vi "MGCC_FntStaMach_Visualization_OpalRT_demo_EvanEdit_v2.vi"() -> ()   [LabVIEW 2016]
panel:
  out "Angle Difference\n0102":dbl format="%#.4f"
  out "Angle Difference\n0405":dbl format="%#.4f"
  out "Angle Difference\n0304":dbl format="%#.4f"
  out "Angle Difference\n0307":dbl format="%#.4f"
  out "Angle Difference\n0709":dbl format="%#.4f"
  out "Angle Difference\n1011":dbl format="%#.4f"
  out "L3":bool
  out "L2":bool
  in  "PV Mode":i32(knob) scale=0.0..2.0
  out "2":cluster{dbl[], dbl[]}(graph)
  out "5":cluster{dbl[], dbl[]}(graph)
  out "4":cluster{dbl[], dbl[]}(graph)
  out "8":cluster{dbl[], dbl[]}(graph)
  out "9":cluster{dbl[], dbl[]}(graph)
  out "11":cluster{dbl[], dbl[]}(graph)
  in  "Stop":bool
  in  "RESET":bool
  out "PV Forecast":dbl[](graph)
  out "3":cluster{dbl[], dbl[]}(graph)
  out "7":cluster{dbl[], dbl[]}(graph)
  out "10":cluster{dbl[], dbl[]}(graph)
  out "13":cluster{dbl[], dbl[]}(graph)
  out "14":cluster{dbl[], dbl[]}(graph)
  out "6":cluster{dbl[], dbl[]}(graph)
  out "1":cluster{dbl[], dbl[]}(graph)
  in  "Tab Control 2":T1(tab)
  out "Loads Power":dbl(graph)
  out "Loads Power":dbl(graph)
  out "Loads Power":dbl(graph)
  out "Loads Power":dbl(graph)
  out "Loads Power":dbl(graph)
  out "Loads Power":dbl(graph)
  out "Loads Power":dbl(graph)
  out "Loads Power":dbl(graph)
  out "Loads Power":dbl(graph)
  in  "Tab Control":T1(tab)
  out "Voltage":dbl(graph)
  out "Voltage":dbl(graph)
  out "Voltage":dbl(graph)
  out "Voltage":dbl(graph)
  out "Voltage":dbl(graph)
  out "Voltage":dbl(graph)
  out "Voltage":dbl(graph)
  out "Voltage":dbl(graph)
  out "Voltage":dbl(graph)
  out "Reactive power control":bool
  out "Active power control":bool
  out "Communication":bool
  out "Reactive power control":bool
  out "Active power control":bool
  out "Resynchronization":bool
  out "Communication":bool
  in  "Island 3":bool
  in  "Island 2":bool
  in  "Island":bool
  in  "Ready for STD":bool
  in  "Recon cmd":bool
  in  "BKS cmd":bool
  in  "island cmd":bool
  out "Angle Difference\n1114":dbl format="%#.4f"
  out "Angle Difference\n0910":dbl format="%#.4f"
  out "Angle Difference\n0406":dbl format="%#.4f"
  out "Angle Difference\n 0203":dbl format="%#.4f"
  out "BESS LC":bool
  out "PV LC":bool
  out "Model Mgmt.":bool
  out "PV Forecasting":bool
  out "Load Forecasting":bool
  out "PQ Balance":bool
  out "Black Start":bool
  out "Data Logging":bool
  out "Communication":bool
  out "State Estimation":bool
  out "Energy Mgmt.":bool
  out "SOC Tank":dbl(slide) scale=0.0..1.0
  out "S1114":bool
  out "S1011":bool
  out "S1012":bool
  out "S1013":bool
  out "S0910":bool
  out "S0708":bool
  out "S0709":bool
  out "S0307":bool
  out "S0304":bool
  out "S0406":bool
  out "S0405":bool
  out "S0203":bool
  out "S0102":bool
  out "W11":bool
  out "W8":bool
  out "L11":bool
  out "W12":bool
  out "L10":bool
  out "L7":bool
  out "L9":bool
  out "W7":bool
  out "L8":bool
  out "L4":bool
  out "L5":bool
  out "W6":bool
  out "W3":bool
  out "W2":bool
  out "Battery Output":dbl format="%#_4f"
  out "Battery SOC":dbl format="%#_4f"
  in  "PV-12":dbl(slide) scale=0.0..2.0
  out "PV Power Output":dbl format="%#_6f"
  out "W4":bool
  out "Current State":string
  out "Sources Power":T2(graph)
  out "Frequency":T3(graph)
  out "W9":bool
  # "Demo: Controller for Flexible Microgrid"
  # "Battery Local Controller"
  # "Microgrid Central\nController"
  # "G-6"
  # "G-14"
  # "G-1"
  # "PV Local Controller"
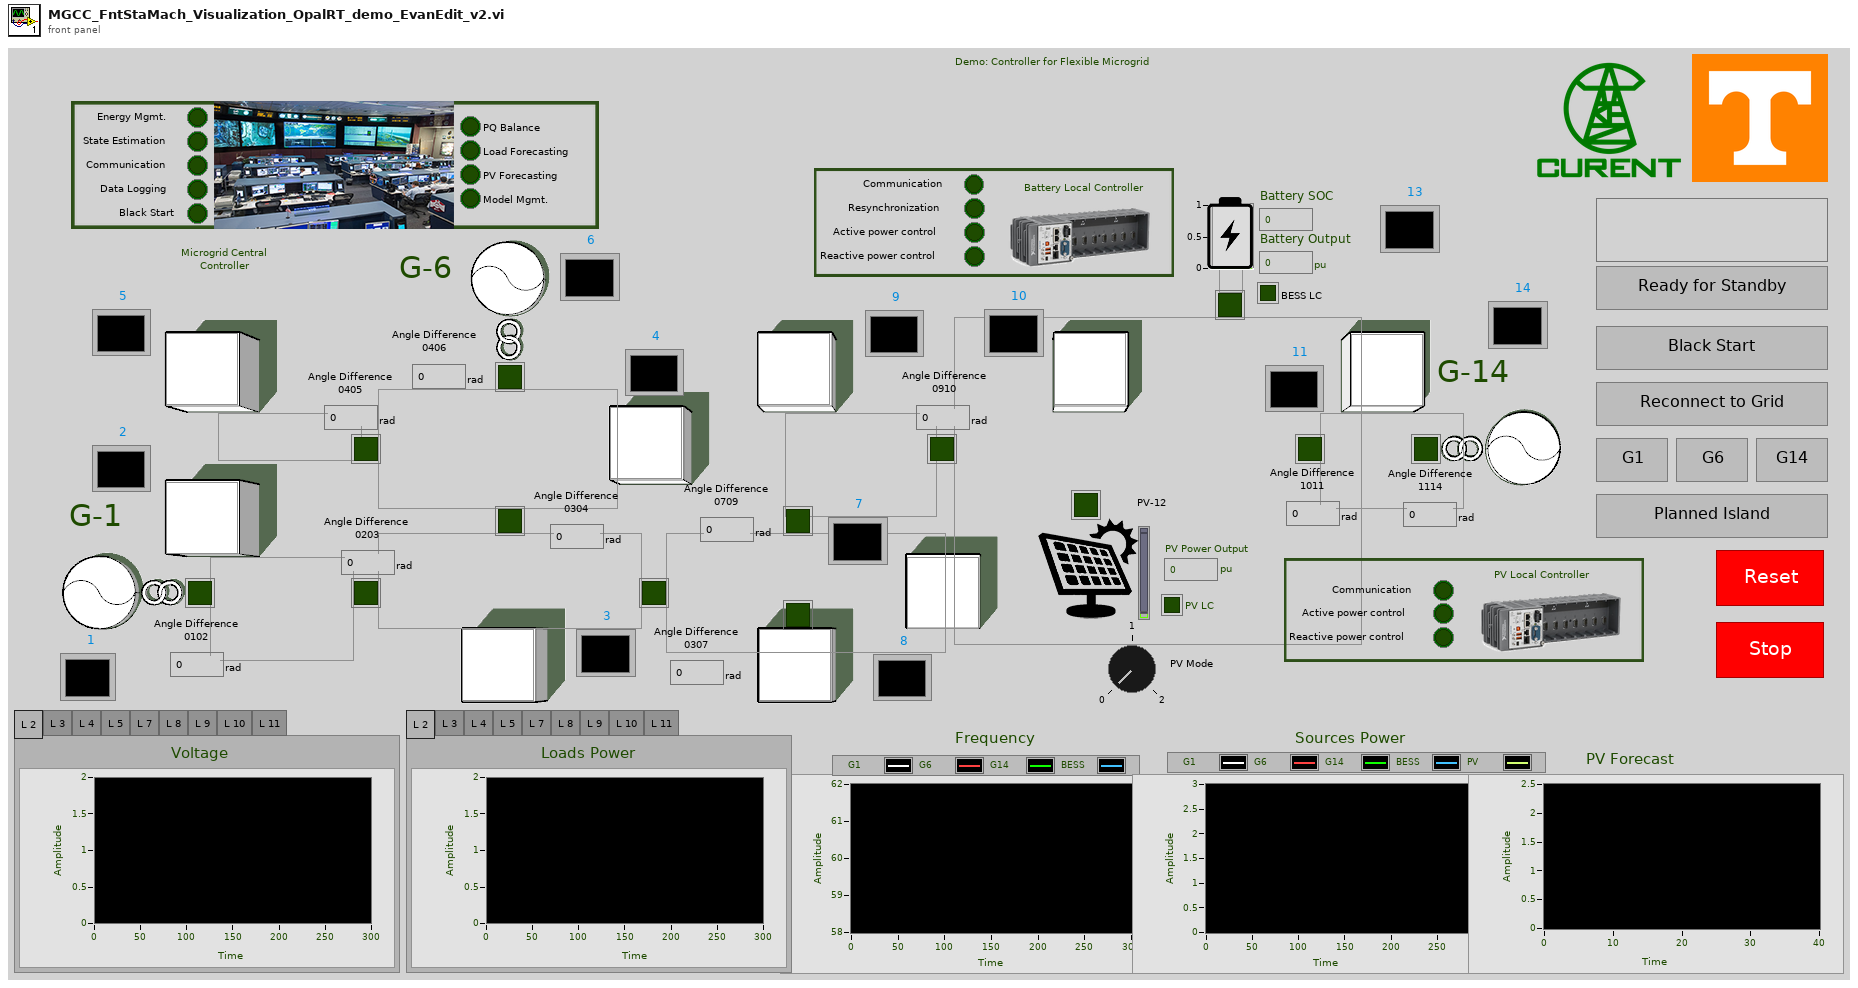
[diagram p1: front panel]
types:
  T1 = enum32{"L 2", "L 3", "L 4", "L 5", "L 7", "L 8", "L 9", "L 10", "L 11"}
  T2 = cluster{"Double":dbl, "Double":dbl, "Double":dbl, "Double":dbl, "Double":dbl}
  T3 = cluster{"Double":dbl, "Double":dbl, "Double":dbl, "Double":dbl}
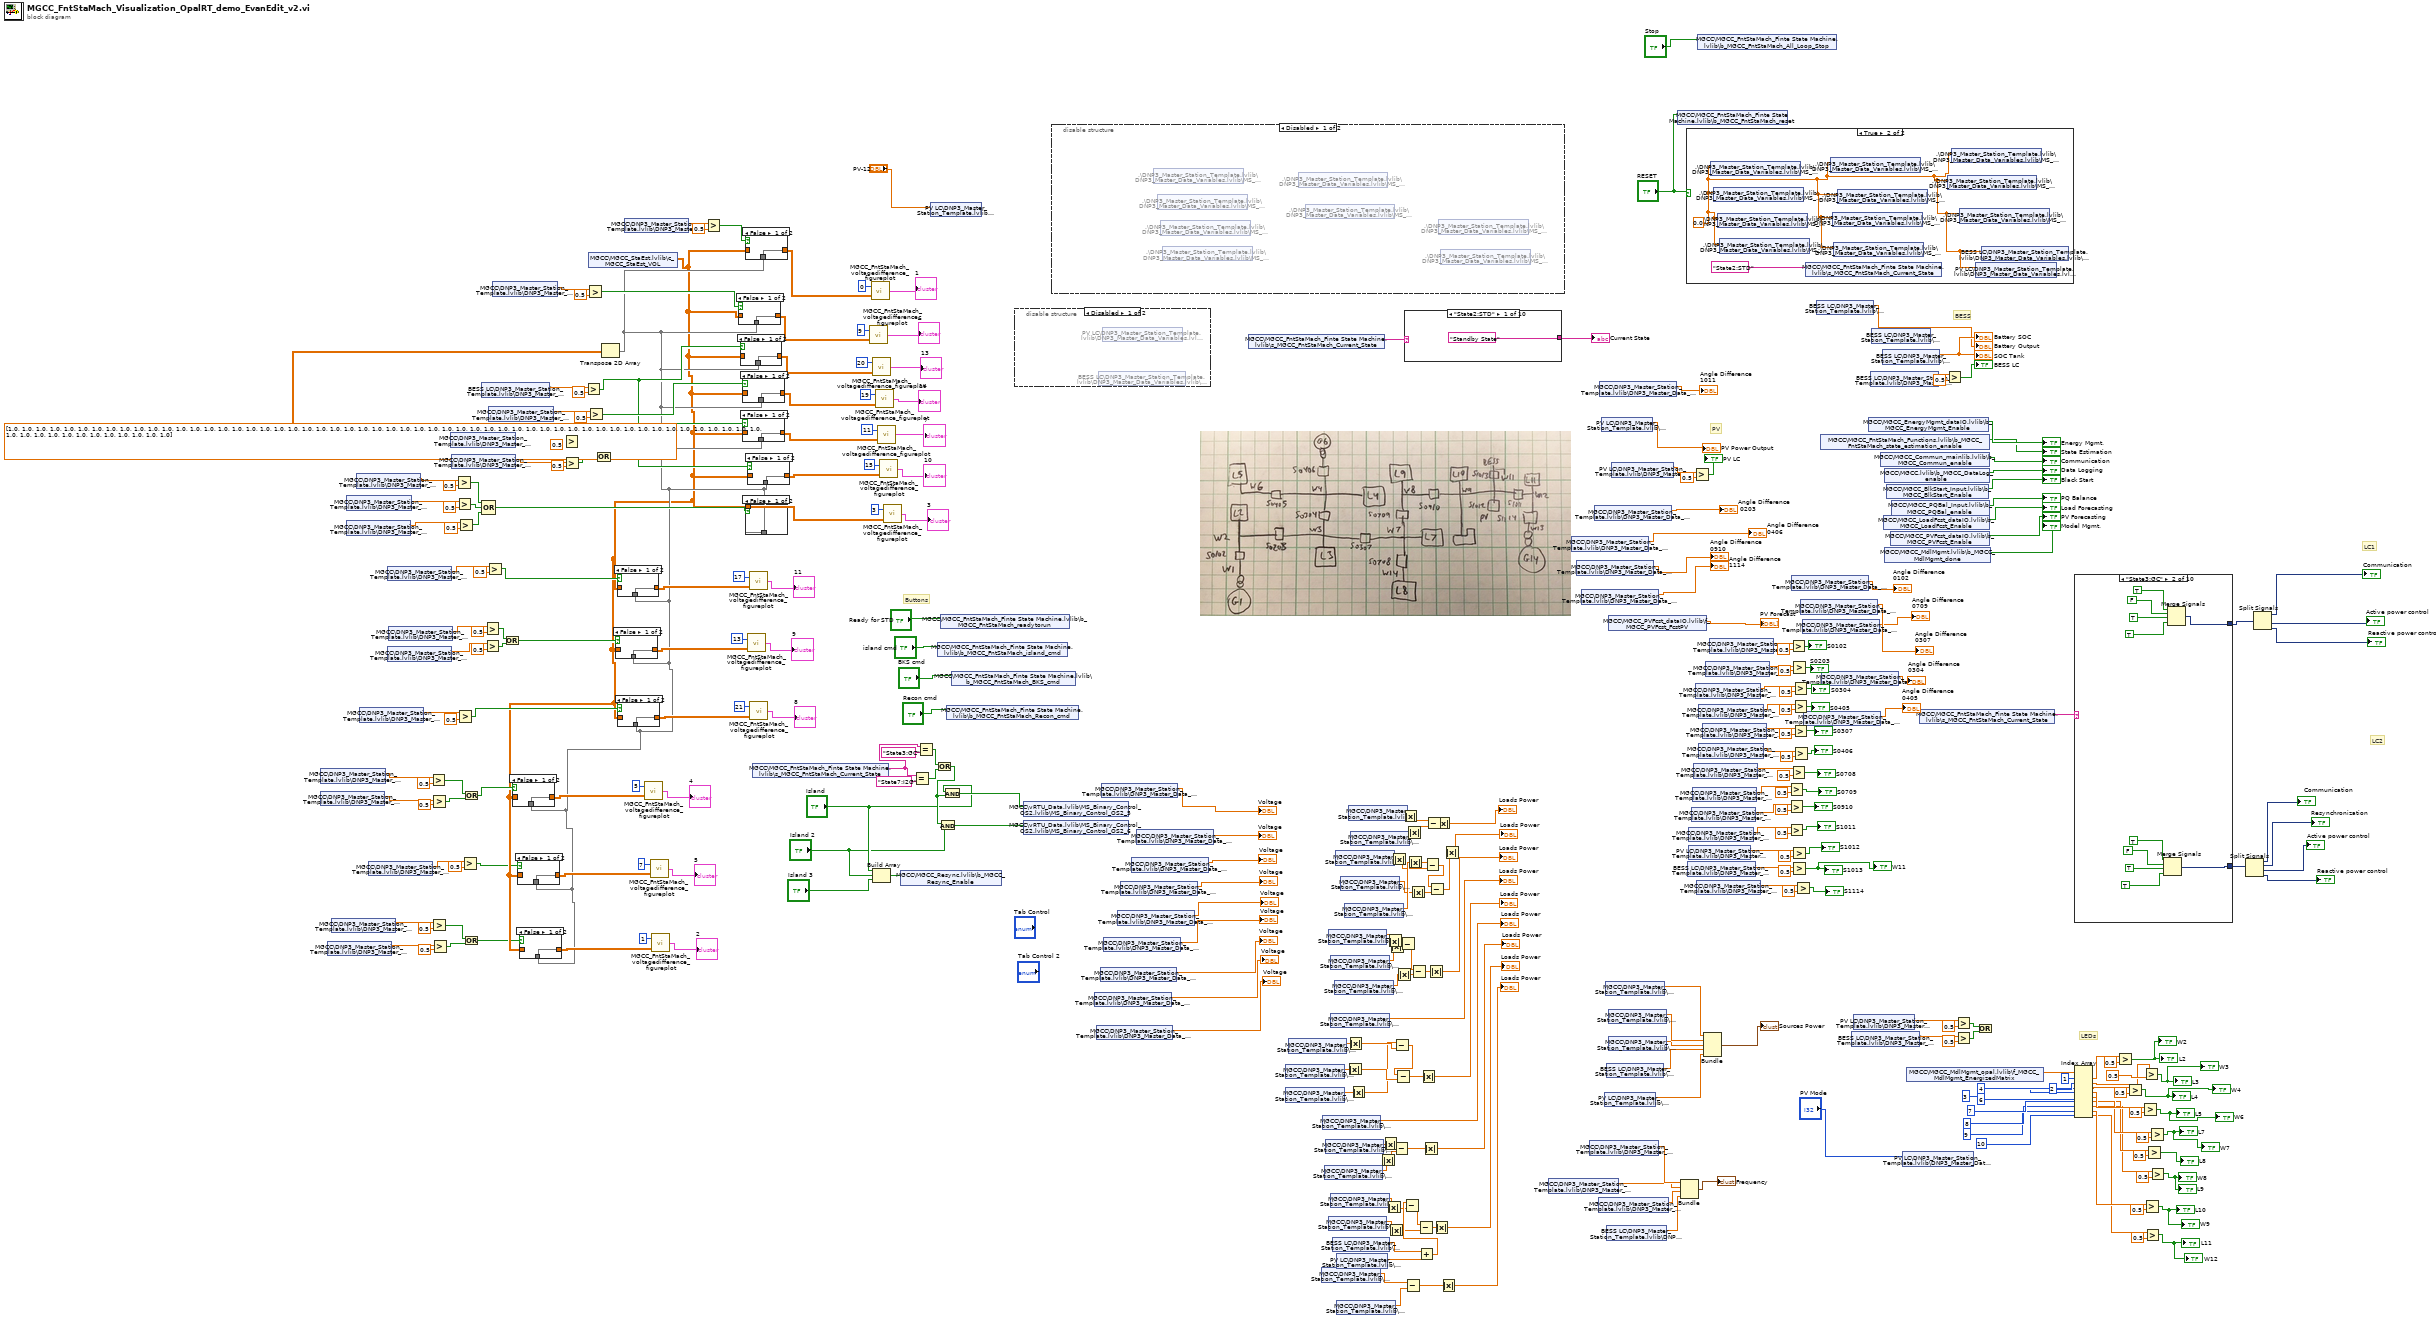
[diagram p0: block diagram]
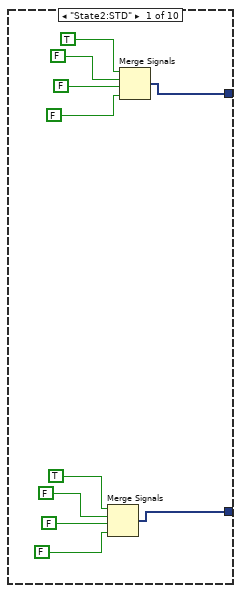
[diagram p2: hidden frame]
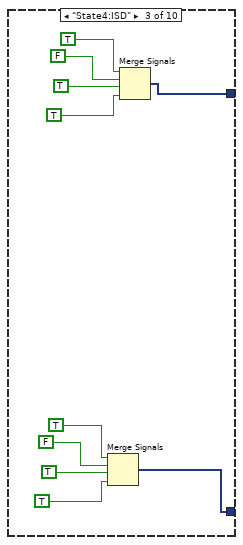
[diagram p3: hidden frame]
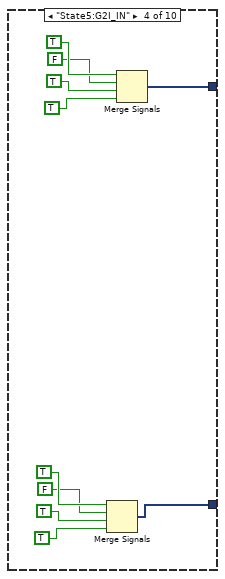
[diagram p4: hidden frame]
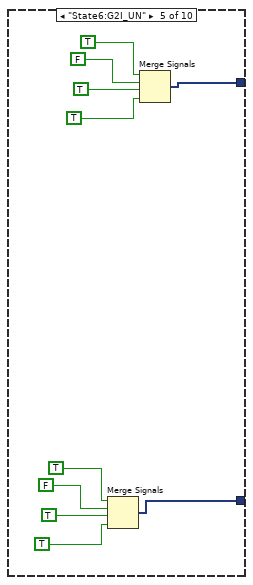
[diagram p5: hidden frame]
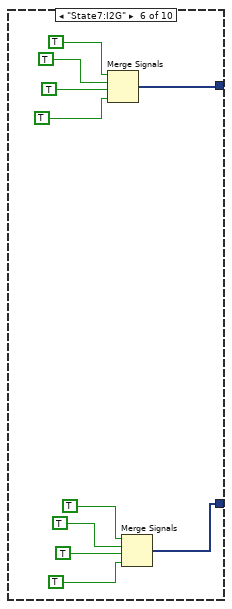
[diagram p6: hidden frame]
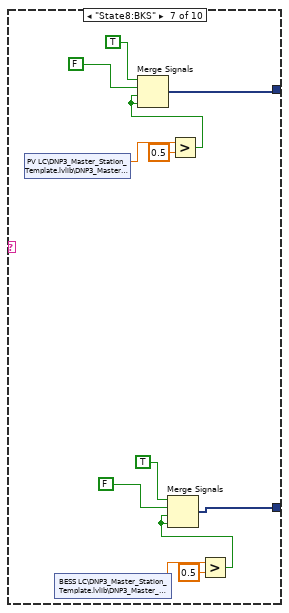
[diagram p7: hidden frame]
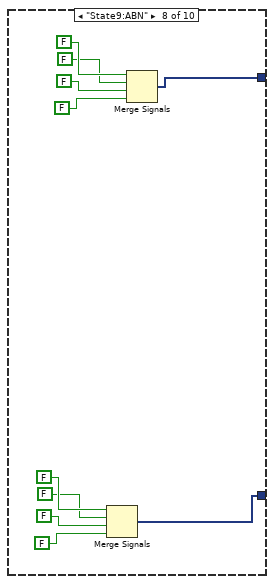
[diagram p8: hidden frame]
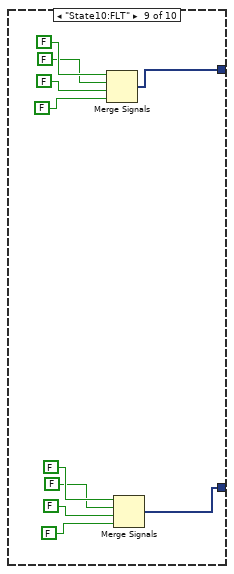
[diagram p9: hidden frame]
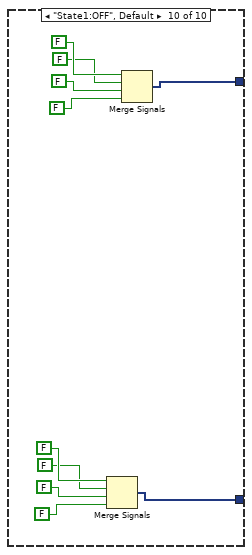
[diagram p10: hidden frame]
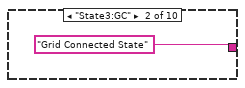
[diagram p18: hidden frame]
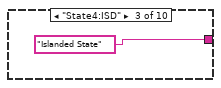
[diagram p19: hidden frame]
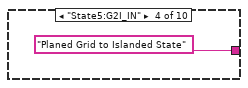
[diagram p20: hidden frame]
diagram:
  # "LC1"
  # "LC2"
  # "PV"
  # "BESS"
  # "Buttons"
  # "LEDs"
  n1 = shared-variable "MGCC\\DNP3_Master_Station_Template.lvlib\\DNP3_Master_Data_Variables.lvlib\\MS_Analog_Status.lvlib\\S0406-status"() -> (w117:dbl)  [unwired: 1 in, 1 out]
  n2 = shared-variable "MGCC\\DNP3_Master_Station_Template.lvlib\\DNP3_Master_Data_Variables.lvlib\\MS_Analog_Status.lvlib\\S0304-status"() -> (w118:dbl)  [unwired: 1 in, 1 out]
  n3 = shared-variable "MGCC\\DNP3_Master_Station_Template.lvlib\\DNP3_Master_Data_Variables.lvlib\\MS_Analog_Status.lvlib\\S0203-status"() -> (w101:dbl)  [unwired: 1 in, 1 out]
  n4 = shared-variable "MGCC\\DNP3_Master_Station_Template.lvlib\\DNP3_Master_Data_Variables.lvlib\\MS_Analog_Status.lvlib\\S0102-status"() -> (w102:dbl)  [unwired: 1 in, 1 out]
  n5 = shared-variable "MGCC\\DNP3_Master_Station_Template.lvlib\\DNP3_Master_Data_Variables.lvlib\\MS_Analog_Status.lvlib\\S0307-status"() -> (w159:dbl)  [unwired: 1 in, 1 out]
  n6 = shared-variable "MGCC\\DNP3_Master_Station_Template.lvlib\\DNP3_Master_Data_Variables.lvlib\\MS_Analog_Status.lvlib\\S0304-status"() -> (w160:dbl)  [unwired: 1 in, 1 out]
  n7 = shared-variable "MGCC\\DNP3_Master_Station_Template.lvlib\\DNP3_Master_Data_Variables.lvlib\\MS_Analog_Status.lvlib\\S0203-status"() -> (w161:dbl)  [unwired: 1 in, 1 out]
  n8 = shared-variable "MGCC\\DNP3_Master_Station_Template.lvlib\\DNP3_Master_Data_Variables.lvlib\\MS_Analog_Status.lvlib\\S0708-status"() -> (w124:dbl)  [unwired: 1 in, 1 out]
  n9 = shared-variable "MGCC\\DNP3_Master_Station_Template.lvlib\\DNP3_Master_Data_Variables.lvlib\\MS_Analog_Status.lvlib\\S0405-status"() -> (w106:dbl)  [unwired: 1 in, 1 out]
  n10 = shared-variable "MGCC\\DNP3_Master_Station_Template.lvlib\\DNP3_Master_Data_Variables.lvlib\\MS_Analog_Status.lvlib\\S1011-status"() -> (w143:dbl)  [unwired: 1 in, 1 out]
  n11 = shared-variable "MGCC\\DNP3_Master_Station_Template.lvlib\\DNP3_Master_Data_Variables.lvlib\\MS_Analog_Status.lvlib\\S0910-status"() -> (w135:dbl)  [unwired: 1 in, 1 out]
  n12 = shared-variable "MGCC\\DNP3_Master_Station_Template.lvlib\\DNP3_Master_Data_Variables.lvlib\\MS_Analog_Status.lvlib\\S0709-status"() -> (w136:dbl)  [unwired: 1 in, 1 out]
  n13 = Greater?(x=w118, y=0.5) -> (0:w120:bool)
  n14 = Greater?(x=w117, y=0.5) -> (0:w119:bool)
  n15 = Greater?(x=w102, y=0.5) -> (0:w100:bool)
  n16 = Greater?(x=w101, y=0.5) -> (0:w99:bool)
  n17 = shared-variable "MGCC\\DNP3_Master_Station_Template.lvlib\\DNP3_Master_Data_Variables.lvlib\\MS_Analog_Status.lvlib\\S0307-status"() -> (w171:dbl)  [unwired: 1 in, 1 out]
  n18 = shared-variable "MGCC\\DNP3_Master_Station_Template.lvlib\\DNP3_Master_Data_Variables.lvlib\\MS_Analog_Status.lvlib\\S0709-status"() -> (w170:dbl)  [unwired: 1 in, 1 out]
  n19 = Greater?(x=w161, y=0.5) -> (0:w158:bool)
  n20 = Greater?(x=w160, y=0.5) -> (0:w157:bool)
  n21 = Greater?(x=w124, y=0.5) -> (0:w123:bool)
  n22 = Greater?(x=w159, y=0.5) -> (0:w156:bool)
  n23 = Greater?(x=w106, y=0.5) -> (0:w105:bool)
  n24 = Or(x=w120, y=w119) -> (x .or. y?=w116:bool)
  n25 = Or(x=w100, y=w99) -> (x .or. y?=w98:bool)
  n26 = shared-variable "BESS LC\\DNP3_Master_Station_Template.lvlib\\DNP3_Master_Data_Variables.lvlib\\MS_Analog_Status.lvlib\\BESS-STATUS"() -> (w183:dbl)  [unwired: 1 in, 1 out]
  n27 = Compound Arithmetic op=OR(w158, w157, w156) -> (w155:bool)
  n28 = Greater?(x=w136, y=0.5) -> (0:w134:bool)
  n29 = Greater?(x=w135, y=0.5) -> (0:w133:bool)
  n30 = Greater?(x=w143, y=0.5) -> (0:w142:bool)
  n31 = shared-variable "MGCC\\DNP3_Master_Station_Template.lvlib\\DNP3_Master_Data_Variables.lvlib\\MS_Analog_Status.lvlib\\S1114-status"() -> (w177:dbl)  [unwired: 1 in, 1 out]
  n32 = shared-variable "MGCC\\DNP3_Master_Station_Template.lvlib\\DNP3_Master_Data_Variables.lvlib\\MS_Analog_Status.lvlib\\S0406-status"() -> (w186:dbl)  [unwired: 1 in, 1 out]
  n33 = Or(x=w134, y=w133) -> (x .or. y?=w132:bool)
  n34 = Greater?(x=w171, y=0.5) -> (0:w173:bool)
  n35 = Greater?(x=w170, y=0.5) -> (0:w172:bool)
  n36 = Greater?(x=w183, y=0.5) -> (0:w168:bool)
  n37 = Greater?(x=w186, y=0.5) -> (0:w185:bool)
  n38 = Greater?(x=w177, y=0.5) -> (0:w176:bool)
  n39 = shared-variable "MGCC\\MGCC_StaEst.lvlib\\c_MGCC_StaEst_VOL"() -> (w108:cdb[][])  [unwired: 1 in, 1 out]
  n40 = Or(x=w173, y=w172) -> (x .or. y?=w169:bool)
  n41 = Transpose 2D Array(2D array=dbl[][] [[1.0, 1.0, 1.0, 1.0, 1.0, 1.0, 1.0, 1.0, 1.0, 1.0, 1.0, 1.0, 1.0, 1.0, 1.0, 1.0, 1.0, 1.0, 1.0, 1.0, 1.0, 1.0], [1.0, 1.0, 1.0, 1.0, 1.0, 1.0, 1.0, 1.0, 1.0, 1.0, 1.0, 1.0, 1.0, 1.0, 1.0, 1.0, 1.0, 1.0, 1.0, 1.0, 1.0, 1.0], [1.0, 1.0, 1.0, 1.0, 1.0, 1.0, 1.0, 1.0, 1.0, 1.0, 1.0, 1.0, 1.0, 1.0, 1.0, 1.0, 1.0, 1.0, 1.0, 1.0, 1.0, 1.0]] ("lower limit")) -> (transposed array=w109:dbl[][])
  n42 = case shown="False" w116 {
    tunnel: w108 -> [_ w321]
    tunnel: [w320 w321] -> w126
    tunnel: w109 -> [w320 _]
    frame False {
    }
    frame True {
    }
  }
  n43 = case shown="False" w105 {
    tunnel: w108 -> [_ w323]
    tunnel: [w322 w323] -> w113
    tunnel: w109 -> [w322 _]
    frame False {
    }
    frame True {
    }
  }
  n44 = case shown="False" w98 {
    tunnel: w108 -> [_ w325]
    tunnel: [w324 w325] -> w110
    tunnel: w109 -> [w324 _]
    frame False {
    }
    frame True {
    }
  }
  n45 = case shown="False" w132 {
    tunnel: w108 -> [_ w327]
    tunnel: [w326 w327] -> w139
    tunnel: w109 -> [w326 _]
    frame False {
    }
    frame True {
    }
  }
  n46 = case shown="False" w142 {
    tunnel: w108 -> [_ w329]
    tunnel: [w328 w329] -> w145
    tunnel: w109 -> [w328 _]
    frame False {
    }
    frame True {
    }
  }
  n47 = case shown="False" w123 {
    tunnel: w108 -> [_ w331]
    tunnel: [w330 w331] -> w129
    tunnel: w109 -> [w330 _]
    frame False {
    }
    frame True {
    }
  }
  n48 = shared-variable "MGCC\\DNP3_Master_Station_Template.lvlib\\DNP3_Master_Data_Variables.lvlib\\MS_Analog_Status.lvlib\\S0102-status"() -> (w190:dbl)  [unwired: 1 in, 1 out]
  n49 = call "MGCC_FntStaMach_voltagedifference_figureplot.vi"("array"=w126, "index (row)"=5) -> ("output cluster"=→"4":cluster{dbl[], dbl[]})
  n50 = call "MGCC_FntStaMach_voltagedifference_figureplot.vi"("array"=w113, "index (row)"=7) -> ("output cluster"=→"5":cluster{dbl[], dbl[]})
  n51 = call "MGCC_FntStaMach_voltagedifference_figureplot.vi"("array"=w110, "index (row)"=1) -> ("output cluster"=→"2":cluster{dbl[], dbl[]})
  n52 = Greater?(x=w190, y=0.5) -> (0:w189:bool)
  n53 = case shown="False" w185 {
    tunnel: w108 -> [_ w333]
    tunnel: [w332 w333] -> w188
    tunnel: w109 -> [w332 _]
    frame False {
    }
    frame True {
    }
  }
  n54 = case shown="False" w168 {
    tunnel: w108 -> [_ w335]
    tunnel: [w334 w335] -> w182
    tunnel: w109 -> [w334 _]
    frame False {
    }
    frame True {
    }
  }
  n55 = case shown="False" w176 {
    tunnel: w108 -> [_ w337]
    tunnel: [w336 w337] -> w181
    tunnel: w109 -> [w336 _]
    frame False {
    }
    frame True {
    }
  }
  n56 = case shown="False" w169 {
    tunnel: w108 -> [_ w339]
    tunnel: [w338 w339] -> w180
    tunnel: w109 -> [w338 _]
    frame False {
    }
    frame True {
    }
  }
  n57 = case shown="False" w189 {
    tunnel: w108 -> [_ w341]
    tunnel: [w340 w341] -> w192
    tunnel: w109 -> [w340 _]
    frame False {
    }
    frame True {
    }
  }
  n58 = case shown="False" w155 {
    tunnel: w108 -> [_ w343]
    tunnel: [w342 w343] -> w165
    tunnel: w109 -> [w342 _]
    frame False {
    }
    frame True {
    }
  }
  n59 = case shown="False" w168 {
    tunnel: w108 -> [_ w345]
    tunnel: [w344 w345] -> w179
    tunnel: w109 -> [w344 _]
    frame False {
    }
    frame True {
    }
  }
  n60 = call "MGCC_FntStaMach_voltagedifference_figureplot.vi"("array"=w139, "index (row)"=13) -> ("output cluster"=→"9":cluster{dbl[], dbl[]})
  n61 = call "MGCC_FntStaMach_voltagedifference_figureplot.vi"("array"=w145, "index (row)"=17) -> ("output cluster"=→"11":cluster{dbl[], dbl[]})
  n62 = call "MGCC_FntStaMach_voltagedifference_figureplot.vi"("array"=w129, "index (row)"=21) -> ("output cluster"=→"8":cluster{dbl[], dbl[]})
  n63 = shared-variable "MGCC\\MGCC_FntStaMach_Finte State Machine.lvlib\\s_MGCC_FntStaMach_Current_State"() -> (w206:string)  [unwired: 1 in, 1 out]
  n64 = call "MGCC_FntStaMach_voltagedifference_figureplot.vi"("array"=w188, "index (row)"=9) -> ("output cluster"=→"6":cluster{dbl[], dbl[]})
  n65 = call "MGCC_FntStaMach_voltagedifference_figureplot.vi"("array"=w192, "index (row)"=0) -> ("output cluster"=→"1":cluster{dbl[], dbl[]})
  n66 = call "MGCC_FntStaMach_voltagedifference_figureplot.vi"("array"=w182, "index (row)"=20) -> ("output cluster"=→"13":cluster{dbl[], dbl[]})
  n67 = Build Array("Island", "Island 2", "Island 3") -> (w79:bool[])
  n68 = call "MGCC_FntStaMach_voltagedifference_figureplot.vi"("array"=w181, "index (row)"=19) -> ("output cluster"=→"14":cluster{dbl[], dbl[]})
  n69 = call "MGCC_FntStaMach_voltagedifference_figureplot.vi"("array"=w180, "index (row)"=11) -> ("output cluster"=→"7":cluster{dbl[], dbl[]})
  n70 = call "MGCC_FntStaMach_voltagedifference_figureplot.vi"("array"=w179, "index (row)"=15) -> ("output cluster"=→"10":cluster{dbl[], dbl[]})
  n71 = call "MGCC_FntStaMach_voltagedifference_figureplot.vi"("array"=w165, "index (row)"=3) -> ("output cluster"=→"3":cluster{dbl[], dbl[]})
  n72 = shared-variable "MGCC\\MGCC_Resync.lvlib\\b_MGCC_Resync_Enable"(w79) -> ()  [unwired: 1 in, 1 out]
  n73 = Equal?(x=w206, y="State7:I2G") -> (x = y?=w297:bool)
  n74 = Equal?(x=w206, y="State3:GC") -> (x = y?=w296:bool)
  n75 = shared-variable "PV LC\\DNP3_Master_Station_Template.lvlib\\DNP3_Master_Data_Variables.lvlib\\MS_Analog_Control.lvlib\\PV-APC"("PV-12") -> ()  [unwired: 1 in, 1 out]
  n76 = Or(x=w296, y=w297) -> (x .or. y?=w295:bool)
  n77 = shared-variable "MGCC\\MGCC_FntStaMach_Finte State Machine.lvlib\\b_MGCC_FntStaMach_island_cmd"("island cmd") -> ()  [unwired: 1 in, 1 out]
  n78 = And(x=w295, y="Island 2") -> (x .and. y?=w293:bool)
  n79 = shared-variable "MGCC\\MGCC_FntStaMach_Finte State Machine.lvlib\\b_MGCC_FntStaMach_readytorun"("Ready for STD") -> ()  [unwired: 1 in, 1 out]
  n80 = And(x="Island", y=w295) -> (x .and. y?=w294:bool)
  n81 = shared-variable "MGCC\\MGCC_FntStaMach_Finte State Machine.lvlib\\b_MGCC_FntStaMach_Recon_cmd"("Recon cmd") -> ()  [unwired: 1 in, 1 out]
  n82 = shared-variable "MGCC\\MGCC_FntStaMach_Finte State Machine.lvlib\\b_MGCC_FntStaMach_BKS_cmd"("BKS cmd") -> ()  [unwired: 1 in, 1 out]
  n83 = disable-structure shown="Disabled" {
    frame Disabled {
      n84 = shared-variable "BESS LC\\DNP3_Master_Station_Template.lvlib\\DNP3_Master_Data_Variables.lvlib\\MS_Analog_Control.lvlib\\BESS-STATUS-CTRL"() -> (w347:dbl)  [unwired: 1 in, 1 out]
      n85 = shared-variable "PV LC\\DNP3_Master_Station_Template.lvlib\\DNP3_Master_Data_Variables.lvlib\\MS_Analog_Control.lvlib\\PV-STATUS-CTRL"() -> (w346:dbl)  [unwired: 1 in, 1 out]
    }
    frame Enabled {
    }
  }
  n86 = shared-variable "MGCC\\vRTU_Data.lvlib\\MS_Binary_Control_OS2.lvlib\\MS_Binary_Control_OS2_5"(w294) -> ()  [unwired: 1 in, 1 out]
  n87 = shared-variable "MGCC\\vRTU_Data.lvlib\\MS_Binary_Control_OS2.lvlib\\MS_Binary_Control_OS2_6"(w293) -> ()  [unwired: 1 in, 1 out]
  n88 = disable-structure shown="Disabled" {
    frame Disabled {
      n89 = shared-variable ".\\DNP3_Master_Station_Template.lvlib\\DNP3_Master_Data_Variables.lvlib\\MS_Analog_Control.lvlib\\S0203-STATUS-CTRL"() -> (w355:dbl)  [unwired: 1 in, 1 out]
      n90 = shared-variable ".\\DNP3_Master_Station_Template.lvlib\\DNP3_Master_Data_Variables.lvlib\\MS_Analog_Control.lvlib\\S0304-STATUS-CTRL"() -> (w354:dbl)  [unwired: 1 in, 1 out]
      n91 = shared-variable ".\\DNP3_Master_Station_Template.lvlib\\DNP3_Master_Data_Variables.lvlib\\MS_Analog_Control.lvlib\\S0307-STATUS-CTRL"() -> (w353:dbl)  [unwired: 1 in, 1 out]
      n92 = shared-variable ".\\DNP3_Master_Station_Template.lvlib\\DNP3_Master_Data_Variables.lvlib\\MS_Analog_Control.lvlib\\S0405-STATUS-CTRL"() -> (w352:dbl)  [unwired: 1 in, 1 out]
      n93 = shared-variable ".\\DNP3_Master_Station_Template.lvlib\\DNP3_Master_Data_Variables.lvlib\\MS_Analog_Control.lvlib\\S0708-STATUS-CTRL"() -> (w351:dbl)  [unwired: 1 in, 1 out]
      n94 = shared-variable ".\\DNP3_Master_Station_Template.lvlib\\DNP3_Master_Data_Variables.lvlib\\MS_Analog_Control.lvlib\\S0709-STATUS-CTRL"() -> (w350:dbl)  [unwired: 1 in, 1 out]
      n95 = shared-variable ".\\DNP3_Master_Station_Template.lvlib\\DNP3_Master_Data_Variables.lvlib\\MS_Analog_Control.lvlib\\S0910-STATUS-CTRL"() -> (w349:dbl)  [unwired: 1 in, 1 out]
      n96 = shared-variable ".\\DNP3_Master_Station_Template.lvlib\\DNP3_Master_Data_Variables.lvlib\\MS_Analog_Control.lvlib\\S1011-STATUS-CTRL"() -> (w348:dbl)  [unwired: 1 in, 1 out]
    }
    frame Enabled {
    }
  }
  n97 = shared-variable "MGCC\\DNP3_Master_Station_Template.lvlib\\DNP3_Master_Data_Variables.lvlib\\MS_Analog_Status.lvlib\\S0910-MAG-A-R"() -> (→"Voltage":dbl)  [unwired: 1 in, 1 out]
  n98 = shared-variable "MGCC\\DNP3_Master_Station_Template.lvlib\\DNP3_Master_Data_Variables.lvlib\\MS_Analog_Status.lvlib\\S1011-MAG-A-R"() -> (→"Voltage":dbl)  [unwired: 1 in, 1 out]
  n99 = shared-variable "MGCC\\DNP3_Master_Station_Template.lvlib\\DNP3_Master_Data_Variables.lvlib\\MS_Analog_Status.lvlib\\S0709-MAG-A-R"() -> (→"Voltage":dbl)  [unwired: 1 in, 1 out]
  n100 = shared-variable "MGCC\\DNP3_Master_Station_Template.lvlib\\DNP3_Master_Data_Variables.lvlib\\MS_Analog_Status.lvlib\\S0102-MAG-A-R"() -> (→"Voltage":dbl)  [unwired: 1 in, 1 out]
  n101 = shared-variable "MGCC\\DNP3_Master_Station_Template.lvlib\\DNP3_Master_Data_Variables.lvlib\\MS_Analog_Status.lvlib\\S0708-MAG-A-R"() -> (→"Voltage":dbl)  [unwired: 1 in, 1 out]
  n102 = shared-variable "MGCC\\DNP3_Master_Station_Template.lvlib\\DNP3_Master_Data_Variables.lvlib\\MS_Analog_Status.lvlib\\S0307-MAG-A-R"() -> (→"Voltage":dbl)  [unwired: 1 in, 1 out]
  n103 = shared-variable "MGCC\\DNP3_Master_Station_Template.lvlib\\DNP3_Master_Data_Variables.lvlib\\MS_Analog_Status.lvlib\\S0405-MAG-A-R"() -> (→"Voltage":dbl)  [unwired: 1 in, 1 out]
  n104 = shared-variable "MGCC\\DNP3_Master_Station_Template.lvlib\\DNP3_Master_Data_Variables.lvlib\\MS_Analog_Status.lvlib\\S0304-MAG-A-R"() -> (→"Voltage":dbl)  [unwired: 1 in, 1 out]
  n105 = shared-variable "MGCC\\DNP3_Master_Station_Template.lvlib\\DNP3_Master_Data_Variables.lvlib\\MS_Analog_Status.lvlib\\S0203-MAG-A-R"() -> (→"Voltage":dbl)  [unwired: 1 in, 1 out]
  n106 = shared-variable "MGCC\\MGCC_FntStaMach_Finte State Machine.lvlib\\s_MGCC_FntStaMach_Current_State"() -> (w152:string)  [unwired: 1 in, 1 out]
  n107 = shared-variable "MGCC\\DNP3_Master_Station_Template.lvlib\\DNP3_Master_Data_Variables.lvlib\\MS_Analog_Status.lvlib\\S0708-APF"() -> (w26:dbl)  [unwired: 1 in, 1 out]
  n108 = shared-variable "MGCC\\DNP3_Master_Station_Template.lvlib\\DNP3_Master_Data_Variables.lvlib\\MS_Analog_Status.lvlib\\S0709-APF"() -> (w28:dbl)  [unwired: 1 in, 1 out]
  n109 = shared-variable "MGCC\\DNP3_Master_Station_Template.lvlib\\DNP3_Master_Data_Variables.lvlib\\MS_Analog_Status.lvlib\\S0307-APF"() -> (w27:dbl)  [unwired: 1 in, 1 out]
  n110 = shared-variable "MGCC\\DNP3_Master_Station_Template.lvlib\\DNP3_Master_Data_Variables.lvlib\\MS_Analog_Status.lvlib\\S1011-APF"() -> (w265:dbl)  [unwired: 1 in, 1 out]
  n111 = shared-variable "MGCC\\DNP3_Master_Station_Template.lvlib\\DNP3_Master_Data_Variables.lvlib\\MS_Analog_Status.lvlib\\S0708-APF"() -> (→"Loads Power":dbl)  [unwired: 1 in, 1 out]
  n112 = shared-variable "MGCC\\DNP3_Master_Station_Template.lvlib\\DNP3_Master_Data_Variables.lvlib\\MS_Analog_Status.lvlib\\S0910-APF"() -> (w268:dbl)  [unwired: 1 in, 1 out]
  n113 = shared-variable "MGCC\\DNP3_Master_Station_Template.lvlib\\DNP3_Master_Data_Variables.lvlib\\MS_Analog_Status.lvlib\\S0709-APF"() -> (w269:dbl)  [unwired: 1 in, 1 out]
  n114 = shared-variable "MGCC\\DNP3_Master_Station_Template.lvlib\\DNP3_Master_Data_Variables.lvlib\\MS_Analog_Status.lvlib\\S0304-APF"() -> (w278:dbl)  [unwired: 1 in, 1 out]
  n115 = shared-variable "MGCC\\DNP3_Master_Station_Template.lvlib\\DNP3_Master_Data_Variables.lvlib\\MS_Analog_Status.lvlib\\S1011-APF"() -> (w11:dbl)  [unwired: 1 in, 1 out]
  n116 = shared-variable "MGCC\\DNP3_Master_Station_Template.lvlib\\DNP3_Master_Data_Variables.lvlib\\MS_Analog_Status.lvlib\\S0405-APF"() -> (w277:dbl)  [unwired: 1 in, 1 out]
  n117 = shared-variable "MGCC\\DNP3_Master_Station_Template.lvlib\\DNP3_Master_Data_Variables.lvlib\\MS_Analog_Status.lvlib\\S0405-APF"() -> (→"Loads Power":dbl)  [unwired: 1 in, 1 out]
  n118 = shared-variable "MGCC\\DNP3_Master_Station_Template.lvlib\\DNP3_Master_Data_Variables.lvlib\\MS_Analog_Status.lvlib\\S0910-APF"() -> (w12:dbl)  [unwired: 1 in, 1 out]
  n119 = shared-variable "BESS LC\\DNP3_Master_Station_Template.lvlib\\DNP3_Master_Data_Variables.lvlib\\MS_Analog_Status.lvlib\\BESS-APO"() -> (w15:dbl)  [unwired: 1 in, 1 out]
  n120 = shared-variable "MGCC\\DNP3_Master_Station_Template.lvlib\\DNP3_Master_Data_Variables.lvlib\\MS_Analog_Status.lvlib\\S0406-APF"() -> (w275:dbl)  [unwired: 1 in, 1 out]
  n121 = shared-variable "MGCC\\DNP3_Master_Station_Template.lvlib\\DNP3_Master_Data_Variables.lvlib\\MS_Analog_Status.lvlib\\S0203-APF"() -> (w36:dbl)  [unwired: 1 in, 1 out]
  n122 = shared-variable "PV LC\\DNP3_Master_Station_Template.lvlib\\DNP3_Master_Data_Variables.lvlib\\MS_Analog_Status.lvlib\\PV-APO"() -> (w14:dbl)  [unwired: 1 in, 1 out]
  n123 = shared-variable "MGCC\\DNP3_Master_Station_Template.lvlib\\DNP3_Master_Data_Variables.lvlib\\MS_Analog_Status.lvlib\\S1114-APF"() -> (w264:dbl)  [unwired: 1 in, 1 out]
  n124 = shared-variable "MGCC\\DNP3_Master_Station_Template.lvlib\\DNP3_Master_Data_Variables.lvlib\\MS_Analog_Status.lvlib\\S0304-APF"() -> (w35:dbl)  [unwired: 1 in, 1 out]
  n125 = shared-variable "MGCC\\DNP3_Master_Station_Template.lvlib\\DNP3_Master_Data_Variables.lvlib\\MS_Analog_Status.lvlib\\S0307-APF"() -> (w37:dbl)  [unwired: 1 in, 1 out]
  n126 = Absolute Value(x=w26) -> (abs(x)=w24:dbl)
  n127 = Absolute Value(x=w27) -> (abs(x)=w25:dbl)
  n128 = shared-variable "MGCC\\DNP3_Master_Station_Template.lvlib\\DNP3_Master_Data_Variables.lvlib\\MS_Analog_Status.lvlib\\S0102-APF"() -> (w283:dbl)  [unwired: 1 in, 1 out]
  n129 = Absolute Value(x=w28) -> (abs(x)=w23:dbl)
  n130 = shared-variable "MGCC\\DNP3_Master_Station_Template.lvlib\\DNP3_Master_Data_Variables.lvlib\\MS_Analog_Status.lvlib\\S0203-APF"() -> (w282:dbl)  [unwired: 1 in, 1 out]
  n131 = Absolute Value(x=w268) -> (abs(x)=w21:dbl)
  n132 = Absolute Value(x=w269) -> (abs(x)=w22:dbl)
  n133 = Absolute Value(x=w12) -> (abs(x)=w10:dbl)
  n134 = Absolute Value(x=w278) -> (abs(x)=w31:dbl)
  n135 = Absolute Value(x=w11) -> (abs(x)=w9:dbl)
  n136 = Absolute Value(x=w277) -> (abs(x)=w30:dbl)
  n137 = Absolute Value(x=w36) -> (abs(x)=w34:dbl)
  n138 = Subtract(x=w22, y=w21) -> (x-y=w267:dbl)
  n139 = Subtract(x=w23, y=w25) -> (x-y=w272:dbl)
  n140 = Subtract(x=w272, y=w24) -> (x-y=w271:dbl)
  n141 = Absolute Value(x=w275) -> (abs(x)=w29:dbl)
  n142 = Subtract(x=w31, y=w30) -> (x-y=w276:dbl)
  n143 = Absolute Value(x=w283) -> (abs(x)=w40:dbl)
  n144 = case shown="\"State2:STD\"" w152 {
    tunnel: ["Standby State" "Grid Connected State" "Islanded State" "Planed Grid to Islanded State" "Unplaned Grid to Islaned State" "Islanded to Grid State" "Black Start State" "Abnormal State" "Fault State" "Off State"] -> w151
    frame "State2:STD" {
    }
    frame "State3:GC" {
    }
    frame "State4:ISD" {
    }
    frame "State5:G2I_IN" {
    }
    frame "State6:G2I_UN" {
    }
    frame "State7:I2G" {
    }
    frame "State8:BKS" {
    }
    frame "State9:ABN" {
    }
    frame "State10:FLT" {
    }
    frame "State1:OFF", Default {
    }
  }
  "Current State" <- w151
  n145 = Subtract(x=w265, y=w264) -> (x-y=w263:dbl)
  n146 = Absolute Value(x=w282) -> (abs(x)=w39:dbl)
  n147 = Absolute Value(x=w37) -> (abs(x)=w33:dbl)
  n148 = Absolute Value(x=w35) -> (abs(x)=w32:dbl)
  n149 = Subtract(x=w276, y=w29) -> (x-y=w274:dbl)
  n150 = Add(x=w15, y=w14) -> (x+y=w13:dbl)
  n151 = Subtract(x=w13, y=w10) -> (x-y=w266:dbl)
  n152 = Subtract(x=w266, y=w9) -> (x-y=w16:dbl)
  n153 = Absolute Value(x=w271) -> (abs(x)=→"Loads Power":dbl)
  n154 = Absolute Value(x=w267) -> (abs(x)=→"Loads Power":dbl)
  n155 = Subtract(x=w33, y=w34) -> (x-y=w280:dbl)
  n156 = Subtract(x=w40, y=w39) -> (x-y=w281:dbl)
  n157 = Absolute Value(x=w274) -> (abs(x)=→"Loads Power":dbl)
  n158 = Subtract(x=w280, y=w32) -> (x-y=w279:dbl)
  n159 = Absolute Value(x=w16) -> (abs(x)=→"Loads Power":dbl)
  n160 = Absolute Value(x=w281) -> (abs(x)=→"Loads Power":dbl)
  n161 = Absolute Value(x=w263) -> (abs(x)=→"Loads Power":dbl)
  n162 = Absolute Value(x=w279) -> (abs(x)=→"Loads Power":dbl)
  n163 = shared-variable "MGCC\\DNP3_Master_Station_Template.lvlib\\DNP3_Master_Data_Variables.lvlib\\MS_Analog_Status.lvlib\\S0406-FREQ-R"() -> (w261:dbl)  [unwired: 1 in, 1 out]
  n164 = shared-variable "MGCC\\DNP3_Master_Station_Template.lvlib\\DNP3_Master_Data_Variables.lvlib\\MS_Analog_Status.lvlib\\S0406-ANG-DIFF"() -> (→"Angle Difference\n0406":dbl)  [unwired: 1 in, 1 out]
  n165 = shared-variable "MGCC\\DNP3_Master_Station_Template.lvlib\\DNP3_Master_Data_Variables.lvlib\\MS_Analog_Status.lvlib\\S0910-ANG-DIFF"() -> (→"Angle Difference\n0910":dbl)  [unwired: 1 in, 1 out]
  n166 = shared-variable "MGCC\\DNP3_Master_Station_Template.lvlib\\DNP3_Master_Data_Variables.lvlib\\MS_Analog_Status.lvlib\\S1114-ANG-DIFF"() -> (→"Angle Difference\n1114":dbl)  [unwired: 1 in, 1 out]
  n167 = shared-variable "MGCC\\DNP3_Master_Station_Template.lvlib\\DNP3_Master_Data_Variables.lvlib\\MS_Analog_Status.lvlib\\S0102-FREQ-L"() -> (w262:dbl)  [unwired: 1 in, 1 out]
  n168 = shared-variable "MGCC\\DNP3_Master_Station_Template.lvlib\\DNP3_Master_Data_Variables.lvlib\\MS_Analog_Status.lvlib\\S0203-ANG-DIFF"() -> (→"Angle Difference\n 0203":dbl)  [unwired: 1 in, 1 out]
  n169 = shared-variable "MGCC\\DNP3_Master_Station_Template.lvlib\\DNP3_Master_Data_Variables.lvlib\\MS_Analog_Status.lvlib\\S1114-FREQ-R"() -> (w260:dbl)  [unwired: 1 in, 1 out]
  n170 = shared-variable "MGCC\\DNP3_Master_Station_Template.lvlib\\DNP3_Master_Data_Variables.lvlib\\MS_Analog_Status.lvlib\\S1011-ANG-DIFF"() -> (→"Angle Difference\n1011":dbl)  [unwired: 1 in, 1 out]
  n171 = shared-variable "PV LC\\DNP3_Master_Station_Template.lvlib\\DNP3_Master_Data_Variables.lvlib\\MS_Analog_Status.lvlib\\PV-APO"() -> (→"PV Power Output":dbl)  [unwired: 1 in, 1 out]
  n172 = shared-variable "PV LC\\DNP3_Master_Station_Template.lvlib\\DNP3_Master_Data_Variables.lvlib\\MS_Analog_Status.lvlib\\PV-APO"() -> (w253:dbl)  [unwired: 1 in, 1 out]
  n173 = shared-variable "MGCC\\DNP3_Master_Station_Template.lvlib\\DNP3_Master_Data_Variables.lvlib\\MS_Analog_Status.lvlib\\S0102-APF"() -> (w257:dbl)  [unwired: 1 in, 1 out]
  n174 = shared-variable "BESS LC\\DNP3_Master_Station_Template.lvlib\\DNP3_Master_Data_Variables.lvlib\\MS_Analog_Status.lvlib\\BESS-APO"() -> (w254:dbl)  [unwired: 1 in, 1 out]
  n175 = shared-variable "BESS LC\\DNP3_Master_Station_Template.lvlib\\DNP3_Master_Data_Variables.lvlib\\MS_Analog_Status.lvlib\\BESS-FREQ"() -> (w259:dbl)  [unwired: 1 in, 1 out]
  n176 = shared-variable "MGCC\\MGCC_PVFcst_dataIO.lvlib\\f_MGCC_PVFcst_FcstPV"() -> (→"PV Forecast":dbl[])  [unwired: 1 in, 1 out]
  n177 = shared-variable "MGCC\\DNP3_Master_Station_Template.lvlib\\DNP3_Master_Data_Variables.lvlib\\MS_Analog_Status.lvlib\\S0406-APF"() -> (w256:dbl)  [unwired: 1 in, 1 out]
  n178 = shared-variable "MGCC\\DNP3_Master_Station_Template.lvlib\\DNP3_Master_Data_Variables.lvlib\\MS_Analog_Status.lvlib\\S1114-APF"() -> (w255:dbl)  [unwired: 1 in, 1 out]
  n179 = shared-variable "PV LC\\DNP3_Master_Station_Template.lvlib\\DNP3_Master_Data_Variables.lvlib\\MS_Analog_Status.lvlib\\PV-STATUS"() -> (w310:dbl)  [unwired: 1 in, 1 out]
  n180 = shared-variable "MGCC\\MGCC_FntStaMach_Finte State Machine.lvlib\\b_MGCC_FntStaMach_reset"("RESET") -> ()  [unwired: 1 in, 1 out]
  n181 = Bundle("Double"=w262, "Double"=w261, "Double"=w260, "Double"=w259) -> (→"Frequency":T3)  [unwired: 1 in]
  n182 = case shown="True" "RESET" {
    frame False {
    }
    frame True {
      w367 = 0.0
      n183 = shared-variable ".\\DNP3_Master_Station_Template.lvlib\\DNP3_Master_Data_Variables.lvlib\\MS_Analog_Control.lvlib\\S0203-STATUS-CTRL"(w367) -> ()  [unwired: 1 in, 1 out]
      n184 = shared-variable ".\\DNP3_Master_Station_Template.lvlib\\DNP3_Master_Data_Variables.lvlib\\MS_Analog_Control.lvlib\\S0304-STATUS-CTRL"(w367) -> ()  [unwired: 1 in, 1 out]
      n185 = shared-variable ".\\DNP3_Master_Station_Template.lvlib\\DNP3_Master_Data_Variables.lvlib\\MS_Analog_Control.lvlib\\S0307-STATUS-CTRL"(w367) -> ()  [unwired: 1 in, 1 out]
      n186 = shared-variable ".\\DNP3_Master_Station_Template.lvlib\\DNP3_Master_Data_Variables.lvlib\\MS_Analog_Control.lvlib\\S0405-STATUS-CTRL"(w367) -> ()  [unwired: 1 in, 1 out]
      n187 = shared-variable "MGCC\\MGCC_FntStaMach_Finte State Machine.lvlib\\s_MGCC_FntStaMach_Current_State"("State2:STD" ("s_MGCC_FntStaMach_Current_State")) -> ()  [unwired: 1 in, 1 out]
      n188 = shared-variable ".\\DNP3_Master_Station_Template.lvlib\\DNP3_Master_Data_Variables.lvlib\\MS_Analog_Control.lvlib\\S0708-STATUS-CTRL"(w367) -> ()  [unwired: 1 in, 1 out]
      n189 = shared-variable ".\\DNP3_Master_Station_Template.lvlib\\DNP3_Master_Data_Variables.lvlib\\MS_Analog_Control.lvlib\\S0910-STATUS-CTRL"(w367) -> ()  [unwired: 1 in, 1 out]
      n190 = shared-variable ".\\DNP3_Master_Station_Template.lvlib\\DNP3_Master_Data_Variables.lvlib\\MS_Analog_Control.lvlib\\S1011-STATUS-CTRL"(w367) -> ()  [unwired: 1 in, 1 out]
      n191 = shared-variable ".\\DNP3_Master_Station_Template.lvlib\\DNP3_Master_Data_Variables.lvlib\\MS_Analog_Control.lvlib\\S0709-STATUS-CTRL"(w367) -> ()  [unwired: 1 in, 1 out]
      n192 = shared-variable ".\\DNP3_Master_Station_Template.lvlib\\DNP3_Master_Data_Variables.lvlib\\MS_Analog_Control.lvlib\\S0406-STATUS-CTRL"(w367) -> ()  [unwired: 1 in, 1 out]
      n193 = shared-variable ".\\DNP3_Master_Station_Template.lvlib\\DNP3_Master_Data_Variables.lvlib\\MS_Analog_Control.lvlib\\S0102-STATUS-CTRL"(w367) -> ()  [unwired: 1 in, 1 out]
      n194 = shared-variable ".\\DNP3_Master_Station_Template.lvlib\\DNP3_Master_Data_Variables.lvlib\\MS_Analog_Control.lvlib\\S1114-STATUS-CTRL"(w367) -> ()  [unwired: 1 in, 1 out]
      n195 = shared-variable "PV LC\\DNP3_Master_Station_Template.lvlib\\DNP3_Master_Data_Variables.lvlib\\MS_Analog_Control.lvlib\\PV-STATUS-CTRL"(w367) -> ()  [unwired: 1 in, 1 out]
      n196 = shared-variable "BESS LC\\DNP3_Master_Station_Template.lvlib\\DNP3_Master_Data_Variables.lvlib\\MS_Analog_Control.lvlib\\BESS-STATUS-CTRL"(w367) -> ()  [unwired: 1 in, 1 out]
    }
  }
  n197 = shared-variable "BESS LC\\DNP3_Master_Station_Template.lvlib\\DNP3_Master_Data_Variables.lvlib\\MS_Analog_Status.lvlib\\BESS-STATUS"() -> (w216:dbl)  [unwired: 1 in, 1 out]
  n198 = shared-variable "MGCC\\DNP3_Master_Station_Template.lvlib\\DNP3_Master_Data_Variables.lvlib\\MS_Analog_Status.lvlib\\S1011-status"() -> (w222:dbl)  [unwired: 1 in, 1 out]
  n199 = shared-variable "PV LC\\DNP3_Master_Station_Template.lvlib\\DNP3_Master_Data_Variables.lvlib\\MS_Analog_Status.lvlib\\PV-STATUS"() -> (w218:dbl)  [unwired: 1 in, 1 out]
  n200 = shared-variable "MGCC\\DNP3_Master_Station_Template.lvlib\\DNP3_Master_Data_Variables.lvlib\\MS_Analog_Status.lvlib\\S0910-status"() -> (w224:dbl)  [unwired: 1 in, 1 out]
  n201 = shared-variable "MGCC\\DNP3_Master_Station_Template.lvlib\\DNP3_Master_Data_Variables.lvlib\\MS_Analog_Status.lvlib\\S0709-status"() -> (w230:dbl)  [unwired: 1 in, 1 out]
  n202 = Greater?(x=w310, y=0.5) -> (0:→"PV LC":bool)
  n203 = shared-variable "MGCC\\DNP3_Master_Station_Template.lvlib\\DNP3_Master_Data_Variables.lvlib\\MS_Analog_Status.lvlib\\S0708-status"() -> (w231:dbl)  [unwired: 1 in, 1 out]
  n204 = shared-variable "MGCC\\DNP3_Master_Station_Template.lvlib\\DNP3_Master_Data_Variables.lvlib\\MS_Analog_Status.lvlib\\S0304-status"() -> (w243:dbl)  [unwired: 1 in, 1 out]
  n205 = shared-variable "MGCC\\DNP3_Master_Station_Template.lvlib\\DNP3_Master_Data_Variables.lvlib\\MS_Analog_Status.lvlib\\S1114-status"() -> (w220:dbl)  [unwired: 1 in, 1 out]
  n206 = shared-variable "MGCC\\MGCC_FntStaMach_Finte State Machine.lvlib\\b_MGCC_FntStaMach_All_Loop_Stop"("Stop") -> ()  [unwired: 1 in, 1 out]
  n207 = shared-variable "MGCC\\DNP3_Master_Station_Template.lvlib\\DNP3_Master_Data_Variables.lvlib\\MS_Analog_Status.lvlib\\S0405-status"() -> (w236:dbl)  [unwired: 1 in, 1 out]
  n208 = shared-variable "MGCC\\DNP3_Master_Station_Template.lvlib\\DNP3_Master_Data_Variables.lvlib\\MS_Analog_Status.lvlib\\S0406-status"() -> (w233:dbl)  [unwired: 1 in, 1 out]
  n209 = shared-variable "MGCC\\DNP3_Master_Station_Template.lvlib\\DNP3_Master_Data_Variables.lvlib\\MS_Analog_Status.lvlib\\S0307-status"() -> (w235:dbl)  [unwired: 1 in, 1 out]
  n210 = Bundle("Double"=w257, "Double"=w256, "Double"=w255, "Double"=w254, "Double"=w253) -> (→"Sources Power":T2)  [unwired: 1 in]
  n211 = shared-variable "MGCC\\DNP3_Master_Station_Template.lvlib\\DNP3_Master_Data_Variables.lvlib\\MS_Analog_Status.lvlib\\S0203-status"() -> (w245:dbl)  [unwired: 1 in, 1 out]
  n212 = shared-variable "MGCC\\DNP3_Master_Station_Template.lvlib\\DNP3_Master_Data_Variables.lvlib\\MS_Analog_Status.lvlib\\S0102-status"() -> (w250:dbl)  [unwired: 1 in, 1 out]
  n213 = Greater?(x=w230, y=0.5) -> (0:→"S0709":bool)
  n214 = Greater?(x=w224, y=0.5) -> (0:→"S0910":bool)
  n215 = Greater?(x=w222, y=0.5) -> (0:→"S1011":bool)
  n216 = Greater?(x=w250, y=0.5) -> (0:→"S0102":bool)
  n217 = Greater?(x=w231, y=0.5) -> (0:→"S0708":bool)
  n218 = Greater?(x=w245, y=0.5) -> (0:→"S0203":bool)
  n219 = Greater?(x=w218, y=0.5) -> (0:→"S1012":bool)
  n220 = Greater?(x=w216, y=0.5) -> (0:→"W11" →"S1013":bool)
  n221 = shared-variable "MGCC\\DNP3_Master_Station_Template.lvlib\\DNP3_Master_Data_Variables.lvlib\\MS_Analog_Status.lvlib\\S0102-ANG-DIFF"() -> (→"Angle Difference\n0102":dbl)  [unwired: 1 in, 1 out]
  n222 = Greater?(x=w243, y=0.5) -> (0:→"S0304":bool)
  n223 = Greater?(x=w236, y=0.5) -> (0:→"S0405":bool)
  n224 = Greater?(x=w235, y=0.5) -> (0:→"S0307":bool)
  n225 = Greater?(x=w233, y=0.5) -> (0:→"S0406":bool)
  n226 = Greater?(x=w220, y=0.5) -> (0:→"S1114":bool)
  n227 = shared-variable "MGCC\\DNP3_Master_Station_Template.lvlib\\DNP3_Master_Data_Variables.lvlib\\MS_Analog_Status.lvlib\\S0307-ANG-DIFF"() -> (→"Angle Difference\n0307":dbl)  [unwired: 1 in, 1 out]
  n228 = shared-variable "MGCC\\DNP3_Master_Station_Template.lvlib\\DNP3_Master_Data_Variables.lvlib\\MS_Analog_Status.lvlib\\S0709-ANG-DIFF"() -> (→"Angle Difference\n0709":dbl)  [unwired: 1 in, 1 out]
  n229 = shared-variable "MGCC\\DNP3_Master_Station_Template.lvlib\\DNP3_Master_Data_Variables.lvlib\\MS_Analog_Status.lvlib\\S0405-ANG-DIFF"() -> (→"Angle Difference\n0405":dbl)  [unwired: 1 in, 1 out]
  n230 = shared-variable "BESS LC\\DNP3_Master_Station_Template.lvlib\\DNP3_Master_Data_Variables.lvlib\\MS_Analog_Status.lvlib\\BESS-APO"() -> (→"Battery Output":dbl)  [unwired: 1 in, 1 out]
  n231 = shared-variable "MGCC\\MGCC_FntStaMach_Functions.lvlib\\b_MGCC_FntStaMach_state_estimation_enable"() -> (→"State Estimation":bool)  [unwired: 1 in, 1 out]
  n232 = shared-variable "MGCC\\DNP3_Master_Station_Template.lvlib\\DNP3_Master_Data_Variables.lvlib\\MS_Analog_Status.lvlib\\S0304-ANG-DIFF"() -> (→"Angle Difference\n0304":dbl)  [unwired: 1 in, 1 out]
  n233 = shared-variable "BESS LC\\DNP3_Master_Station_Template.lvlib\\DNP3_Master_Data_Variables.lvlib\\MS_Analog_Status.lvlib\\BESS-STATUS"() -> (w210:dbl)  [unwired: 1 in, 1 out]
  n234 = shared-variable "PV LC\\DNP3_Master_Station_Template.lvlib\\DNP3_Master_Data_Variables.lvlib\\MS_Analog_Status.lvlib\\PV-STATUS"() -> (w211:dbl)  [unwired: 1 in, 1 out]
  n235 = shared-variable "MGCC\\MGCC_EnergyMgmt_dataIO.lvlib\\b_MGCC_EnergyMgmt_Enable"() -> (→"Energy Mgmt.":bool)  [unwired: 1 in, 1 out]
  n236 = shared-variable "BESS LC\\DNP3_Master_Station_Template.lvlib\\DNP3_Master_Data_Variables.lvlib\\MS_Analog_Status.lvlib\\BESS-STATUS"() -> (w314:dbl)  [unwired: 1 in, 1 out]
  n237 = shared-variable "BESS LC\\DNP3_Master_Station_Template.lvlib\\DNP3_Master_Data_Variables.lvlib\\MS_Analog_Status.lvlib\\BESS-MAG"() -> ()  [unwired: 1 in, 2 out]
  n238 = shared-variable "MGCC\\MGCC_Commun_mainlib.lvlib\\b_MGCC_Commun_enable"() -> (→"Communication":bool)  [unwired: 1 in, 1 out]
  n239 = shared-variable "BESS LC\\DNP3_Master_Station_Template.lvlib\\DNP3_Master_Data_Variables.lvlib\\MS_Analog_Status.lvlib\\BESS-SOC"() -> (→"Battery SOC" →"SOC Tank":dbl)  [unwired: 1 in, 1 out]
  n240 = shared-variable "MGCC\\MGCC_LoadFcst_dataIO.lvlib\\b_MGCC_LoadFcst_Enable"() -> (→"Load Forecasting":bool)  [unwired: 1 in, 1 out]
  n241 = shared-variable "MGCC\\MGCC.lvlib\\b_MGCC_DataLog_enable"() -> (→"Data Logging":bool)  [unwired: 1 in, 1 out]
  n242 = shared-variable "MGCC\\MGCC_MdlMgmt.lvlib\\b_MGCC_MdlMgmt_done"() -> (→"Model Mgmt.":bool)  [unwired: 1 in, 1 out]
  n243 = shared-variable "MGCC\\MGCC_BlkStart_Input.lvlib\\b_MGCC_BlkStart_Enable"() -> (→"Black Start":bool)  [unwired: 1 in, 1 out]
  n244 = shared-variable "MGCC\\MGCC_PVFcst_dataIO.lvlib\\b_MGCC_PVFcst_Enable"() -> (→"PV Forecasting":bool)  [unwired: 1 in, 1 out]
  n245 = shared-variable "MGCC\\MGCC_PQBal_Input.lvlib\\b_MGCC_PQBal_enable"() -> (→"PQ Balance":bool)  [unwired: 1 in, 1 out]
  n246 = shared-variable "PV LC\\DNP3_Master_Station_Template.lvlib\\DNP3_Master_Data_Variables.lvlib\\MS_Analog_Control.lvlib\\PV-RESERVED4"("PV Mode") -> ()  [unwired: 1 in, 1 out]
  n247 = shared-variable "MGCC\\MGCC_MdlMgmt_opal.lvlib\\f_MGCC_MdlMgmt_EnergizedMatrix"() -> (w78:dbl[])  [unwired: 1 in, 1 out]
  n248 = shared-variable "MGCC\\MGCC_FntStaMach_Finte State Machine.lvlib\\s_MGCC_FntStaMach_Current_State"() -> (w92:string)  [unwired: 1 in, 1 out]
  n249 = Greater?(x=w314, y=0.5) -> (0:→"BESS LC":bool)
  n250 = Greater?(x=w211, y=0.5) -> (0:w209:bool)
  n251 = Greater?(x=w210, y=0.5) -> (0:w208:bool)
  n252 = Or(x=w209, y=w208) -> ()  [unwired: 1 out]
  n253 = Index Array(array=w78, index #1=1 ("index"), index #2=2 ("index"), index #3=3 ("index"), index #4=4 ("index"), index #5=6 ("index"), index #6=7 ("index"), index #7=8 ("index"), index #8=9 ("index"), index #9=10 ("index")) -> (element #1=w75:dbl, element #2=w72:dbl, element #3=w69:dbl, element #4=w66:dbl, element #5=w63:dbl, element #6=w55:dbl, element #7=w50:dbl, element #8=w47:dbl, element #9=w43:dbl)
  n254 = case shown="\"State3:GC\"" w92 {
    tunnel: [w373 w383 w393 w403 w413 w426 w438 w445 w455 w465] -> w91
    tunnel: [w368 w379 w389 w398 w408 w418 w428 w440 w450 w460] -> w87
    frame "State2:STD" {
      n255 = Merge Signals(TRUE ("Resynchronization"), FALSE ("Resynchronization"), FALSE ("Resynchronization"), FALSE ("Resynchronization")) -> (w368:dynamicdata)
      n256 = Merge Signals(TRUE ("Resynchronization"), FALSE ("Resynchronization"), FALSE ("Resynchronization"), FALSE ("Resynchronization")) -> (w373:dynamicdata)
    }
    frame "State3:GC" {
      n257 = Merge Signals(TRUE ("Resynchronization"), FALSE ("Resynchronization"), TRUE ("Resynchronization"), TRUE ("Resynchronization")) -> (w379:dynamicdata)
      n258 = Merge Signals(TRUE ("Resynchronization"), FALSE ("Resynchronization"), TRUE ("Resynchronization"), TRUE ("Resynchronization")) -> (w383:dynamicdata)
    }
    frame "State4:ISD" {
      n259 = Merge Signals(TRUE ("Resynchronization"), FALSE ("Resynchronization"), TRUE ("Resynchronization"), TRUE ("Resynchronization")) -> (w389:dynamicdata)
      n260 = Merge Signals(TRUE ("Resynchronization"), FALSE ("Resynchronization"), TRUE ("Resynchronization"), TRUE ("Resynchronization")) -> (w393:dynamicdata)
    }
    frame "State5:G2I_IN" {
      n261 = Merge Signals(TRUE ("Resynchronization"), FALSE ("Resynchronization"), TRUE ("Resynchronization"), TRUE ("Resynchronization")) -> (w398:dynamicdata)
      n262 = Merge Signals(TRUE ("Resynchronization"), FALSE ("Resynchronization"), TRUE ("Resynchronization"), TRUE ("Resynchronization")) -> (w403:dynamicdata)
    }
    frame "State6:G2I_UN" {
      n263 = Merge Signals(TRUE ("Resynchronization"), FALSE ("Resynchronization"), TRUE ("Resynchronization"), TRUE ("Resynchronization")) -> (w408:dynamicdata)
      n264 = Merge Signals(TRUE ("Resynchronization"), FALSE ("Resynchronization"), TRUE ("Resynchronization"), TRUE ("Resynchronization")) -> (w413:dynamicdata)
    }
    frame "State7:I2G" {
      n265 = Merge Signals(TRUE ("Resynchronization"), TRUE ("Resynchronization"), TRUE ("Resynchronization"), TRUE ("Resynchronization")) -> (w426:dynamicdata)
      n266 = Merge Signals(TRUE ("Resynchronization"), TRUE ("Resynchronization"), TRUE ("Resynchronization"), TRUE ("Resynchronization")) -> (w418:dynamicdata)
    }
    frame "State8:BKS" {
      n267 = shared-variable "PV LC\\DNP3_Master_Station_Template.lvlib\\DNP3_Master_Data_Variables.lvlib\\MS_Analog_Status.lvlib\\PV-STATUS"() -> (w437:dbl)  [unwired: 1 in, 1 out]
      n268 = shared-variable "BESS LC\\DNP3_Master_Station_Template.lvlib\\DNP3_Master_Data_Variables.lvlib\\MS_Analog_Status.lvlib\\BESS-STATUS"() -> (w432:dbl)  [unwired: 1 in, 1 out]
      n269 = Greater?(x=w437, y=0.5) -> (0:w435:bool)
      n270 = Merge Signals(TRUE ("Resynchronization"), FALSE ("Resynchronization"), w435, w435) -> (w438:dynamicdata)
      n271 = Greater?(x=w432, y=0.5) -> (0:w430:bool)
      n272 = Merge Signals(TRUE ("Resynchronization"), FALSE ("Resynchronization"), w430, w430) -> (w428:dynamicdata)
    }
    frame "State9:ABN" {
      n273 = Merge Signals(FALSE ("Resynchronization"), FALSE ("Resynchronization"), FALSE ("Resynchronization"), FALSE ("Resynchronization")) -> (w440:dynamicdata)
      n274 = Merge Signals(FALSE ("Resynchronization"), FALSE ("Resynchronization"), FALSE ("Resynchronization"), FALSE ("Resynchronization")) -> (w445:dynamicdata)
    }
    frame "State10:FLT" {
      n275 = Merge Signals(FALSE ("Resynchronization"), FALSE ("Resynchronization"), FALSE ("Resynchronization"), FALSE ("Resynchronization")) -> (w455:dynamicdata)
      n276 = Merge Signals(FALSE ("Resynchronization"), FALSE ("Resynchronization"), FALSE ("Resynchronization"), FALSE ("Resynchronization")) -> (w450:dynamicdata)
    }
    frame "State1:OFF", Default {
      n277 = Merge Signals(FALSE ("Resynchronization"), FALSE ("Resynchronization"), FALSE ("Resynchronization"), FALSE ("Resynchronization")) -> (w460:dynamicdata)
      n278 = Merge Signals(FALSE ("Resynchronization"), FALSE ("Resynchronization"), FALSE ("Resynchronization"), FALSE ("Resynchronization")) -> (w465:dynamicdata)
    }
  }
  n279 = Greater?(x=w75, y=0.5) -> (0:→"W2" →"L2":bool)
  n280 = Greater?(x=w69, y=0.5) -> (0:→"W4" →"L4":bool)
  n281 = Greater?(x=w66, y=0.5) -> (0:→"W6" →"L5":bool)
  n282 = Greater?(x=w72, y=0.5) -> (0:→"W3" →"L3":bool)
  n283 = Greater?(x=w47, y=0.5) -> (0:→"L10" →"W9":bool)
  n284 = Greater?(x=w43, y=0.5) -> (0:→"W12" →"L11":bool)
  n285 = Greater?(x=w55, y=0.5) -> (0:→"L8":bool)
  n286 = Greater?(x=w63, y=0.5) -> (0:→"W7" →"L7":bool)
  n287 = Greater?(x=w50, y=0.5) -> (0:→"L9" →"W8":bool)
  n288 = Split Signals(w87) -> (→"Communication":dynamicdata, →"Resynchronization":dynamicdata, →"Active power control":dynamicdata, →"Reactive power control":dynamicdata)  [unwired: 4 in]
  n289 = Split Signals(w91) -> (→"Communication":dynamicdata, →"Active power control":dynamicdata, →"Reactive power control":dynamicdata)  [unwired: 4 in, 1 out]
